vi "AIT 1553 - Create BC Message Name.vi"(0 "BC_Message":T1={"Name"="Gun Control", "Tx-Rx_T-Tx"=FALSE, "RT_Address"=11, "RT_SA_Address"=10, "Parameters"=[], "Transfer Enabled"=FALSE, "Message Buffer ID"=30, "Default_Message_Buffer_Data"=[], "Word_Count"=0}, 11 "error in (no error)":errorcluster) -> (4 "Message Name":string="CB_R_A_1E_Gun Control", 15 "error out":errorcluster)   [LabVIEW 2013, in "AIT 1553 Custom Device.lvlib"]
uses:
  AIT 1553 Custom Device.lvlib
  Controls/1553_BC_Message.ctl
  Controls/1553 Param.ctl
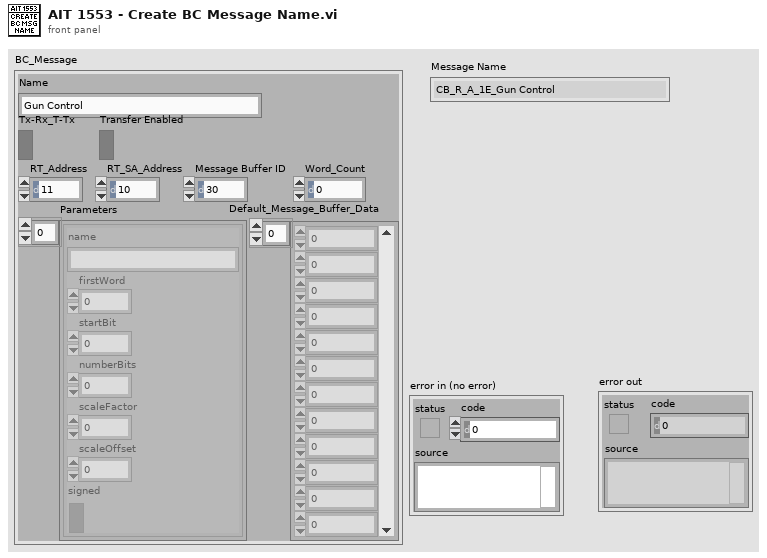
[diagram p1: front panel]
types:
  T1 = typedef "AIT 1553 Custom Device.lvlib/1553_BC_Message.ctl" = cluster{"Name":string, "Tx-Rx_T-Tx":bool, "RT_Address":u8, "RT_SA_Address":u8, "Parameters":T2[], "Transfer Enabled":bool, "Message Buffer ID":u16, "Default_Message_Buffer_Data":u16[], "Word_Count":u8}
  T2 = typedef "AIT 1553 Custom Device.lvlib/1553 Param.ctl" = cluster{"name":string, "firstWord":i32, "startBit":i32, "numberBits":i32, "scaleFactor":dbl, "scaleOffset":dbl, "signed":bool}
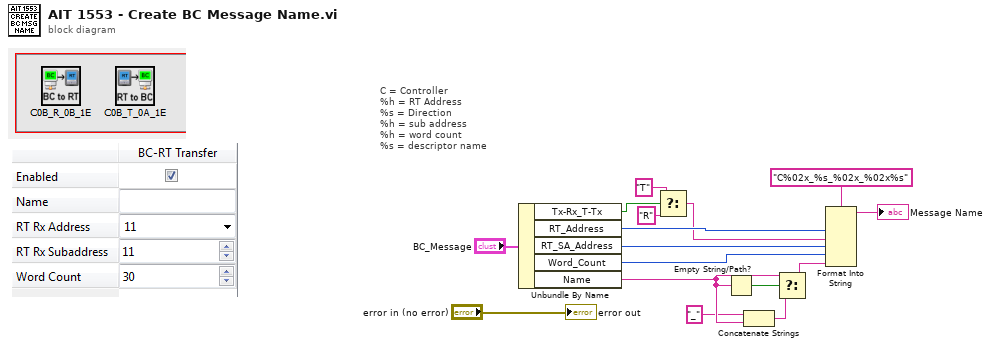
[diagram p0: block diagram]
diagram:
  # "C = Controller\n%h = RT Address\n%s = Direction\n%h = sub address\n%h = word count\n%s = descriptor name"
  n1 = Unbundle By Name("BC_Message") -> ("Tx-Rx_T-Tx"=w13:bool, "RT_Address"=w14:u8, "RT_SA_Address"=w9:u8, "Word_Count"=w1:u8, "Name"=w5:string)
  n2 = Select(t="T", s=w13, f="R") -> (s? t:f=w10:string)
  n3 = Empty String/Path?(string/path=w5) -> (empty?=w6:bool)
  n4 = Concatenate Strings("_" ("string"), w5) -> (w3:string)
  n5 = Select(t=w5, s=w6, f=w3) -> (s? t:f=w2:string)
  n6 = Format Into String(format string="C%02x_%s_%02x_%02x%s", w14, w10, w9, w1, w2) -> (resulting string=→"Message Name":string)  [unwired: 2 in, 1 out]
  "error out" <- "error in (no error)"
